vi "HVppSequence.vi"() -> ()   [LabVIEW 2013]
panel:
  in  "Number of seconds for \neach HVpp case state":dbl=30.0
  out "Elapsed Time (s)":dbl
  in  "?":bool
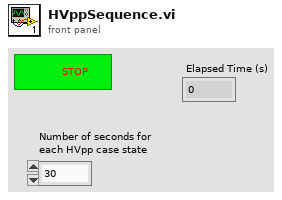
[diagram p1: front panel]
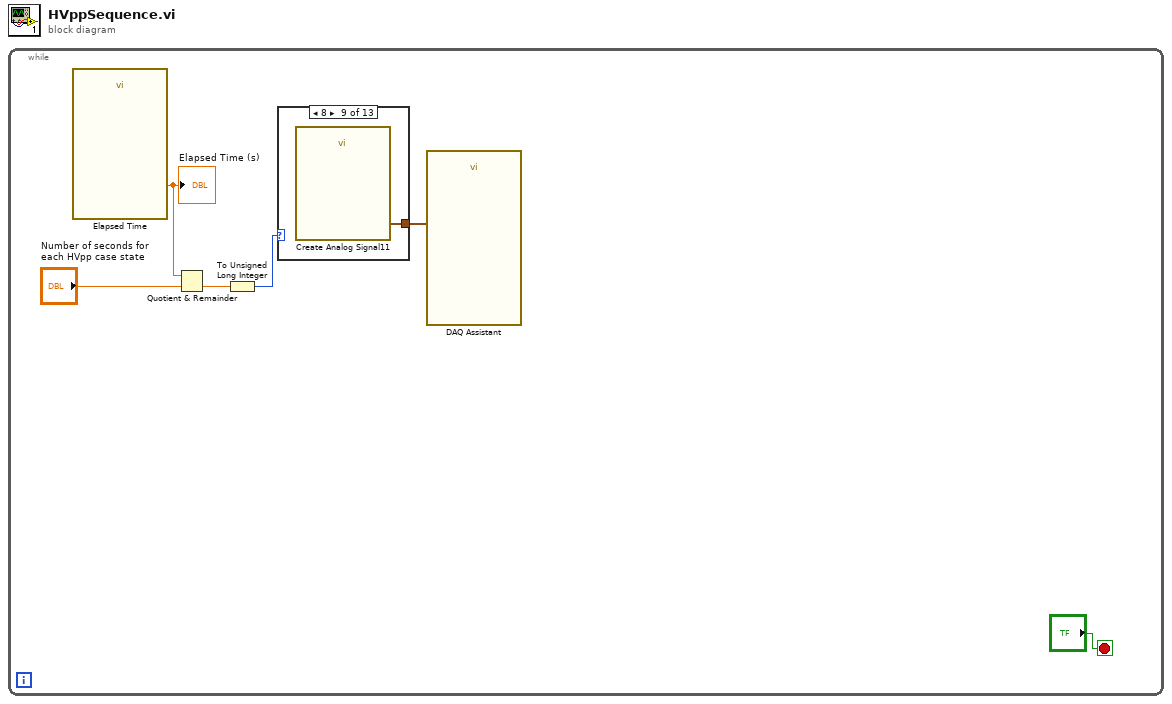
[diagram p0: block diagram]
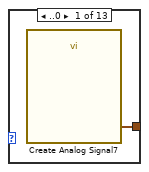
[diagram p2: hidden frame]
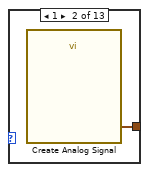
[diagram p3: hidden frame]
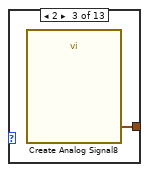
[diagram p4: hidden frame]
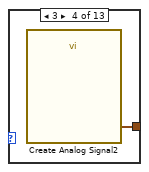
[diagram p5: hidden frame]
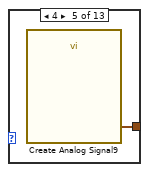
[diagram p6: hidden frame]
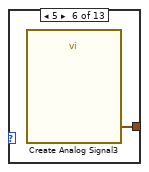
[diagram p7: hidden frame]
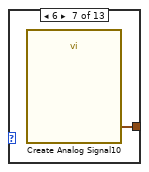
[diagram p8: hidden frame]
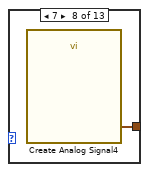
[diagram p9: hidden frame]
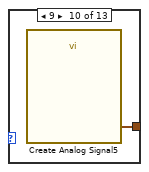
[diagram p10: hidden frame]
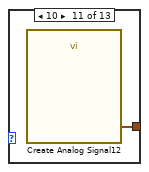
[diagram p11: hidden frame]
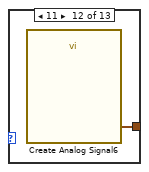
[diagram p12: hidden frame]
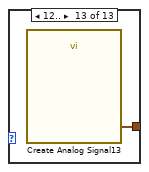
[diagram p13: hidden frame]
diagram:
  n1 = while {
    stop <- "?" stop-if-true
    n2 = call "Elapsed Time"() -> ("Elapsed Time (s)"=w2:dbl)  [unwired: 12 in, 7 out]
    "Elapsed Time (s)" <- w2
    n3 = Quotient & Remainder(x=w2, y="Number of seconds for \neach HVpp case state") -> (floor(x/y)=w3:dbl)  [unwired: 1 out]
    n4 = To Unsigned Long Integer(number=w3) -> (unsigned 32bit integer=w4:u32)
    n5 = case shown="8" w4 {
      tunnel: [w7 w8 w9 w10 w11 w12 w13 w14 w15 w16 w17 w18 w19] -> w5
      frame ..0 {
        n6 = call "Create Analog Signal7"() -> ("sine wave"=w7:waveform(dbl))  [unwired: 18 in, 1 out]
      }
      frame 1 {
        n7 = call "Create Analog Signal"() -> ("sine wave"=w8:waveform(dbl))  [unwired: 18 in, 1 out]
      }
      frame 2 {
        n8 = call "Create Analog Signal8"() -> ("sine wave"=w9:waveform(dbl))  [unwired: 18 in, 1 out]
      }
      frame 3 {
        n9 = call "Create Analog Signal2"() -> ("sine wave"=w10:waveform(dbl))  [unwired: 18 in, 1 out]
      }
      frame 4 {
        n10 = call "Create Analog Signal9"() -> ("sine wave"=w11:waveform(dbl))  [unwired: 18 in, 1 out]
      }
      frame 5 {
        n11 = call "Create Analog Signal3"() -> ("sine wave"=w12:waveform(dbl))  [unwired: 18 in, 1 out]
      }
      frame 6 {
        n12 = call "Create Analog Signal10"() -> ("sine wave"=w13:waveform(dbl))  [unwired: 18 in, 1 out]
      }
      frame 7 {
        n13 = call "Create Analog Signal4"() -> ("sine wave"=w14:waveform(dbl))  [unwired: 18 in, 1 out]
      }
      frame 8 {
        n14 = call "Create Analog Signal11"() -> ("sine wave"=w15:waveform(dbl))  [unwired: 18 in, 1 out]
      }
      frame 9 {
        n15 = call "Create Analog Signal5"() -> ("sine wave"=w16:waveform(dbl))  [unwired: 18 in, 1 out]
      }
      frame 10 {
        n16 = call "Create Analog Signal12"() -> ("sine wave"=w17:waveform(dbl))  [unwired: 18 in, 1 out]
      }
      frame 11 {
        n17 = call "Create Analog Signal6"() -> ("sine wave"=w18:waveform(dbl))  [unwired: 18 in, 1 out]
      }
      frame 12.. {
        n18 = call "Create Analog Signal13"() -> ("sine wave"=w19:waveform(dbl))  [unwired: 18 in, 1 out]
      }
    }
    n19 = call "DAQ Assistant"("data"=w5) -> ()  [unwired: 16 in, 3 out]
  }
